vi "SN3218 Example.vi"() -> ()   [LabVIEW 2020]
uses:
  <vilib>/MakerHub/LINX/Public/Utilities/Open Local.vi
  LINX I2C/LINX I2C.lvclass
  LINX-SN3218/LINX-SN3218.lvclass
  <vilib>/MakerHub/LINX/LMH-LINX.lvlib
panel:
  in  "Channel Output":u8(slide) scale=0.0..255.0
  in  "LED Channel (0-18, 0=all)":u8
  in  "Enabled?":bool[](array[boolean])=[FALSE, FALSE, FALSE, FALSE, FALSE, FALSE, FALSE, FALSE, FALSE, FALSE, FALSE, FALSE, FALSE, FALSE, FALSE, FALSE, FALSE, FALSE]
  in  "stop":bool
  out "Error Out":errorcluster
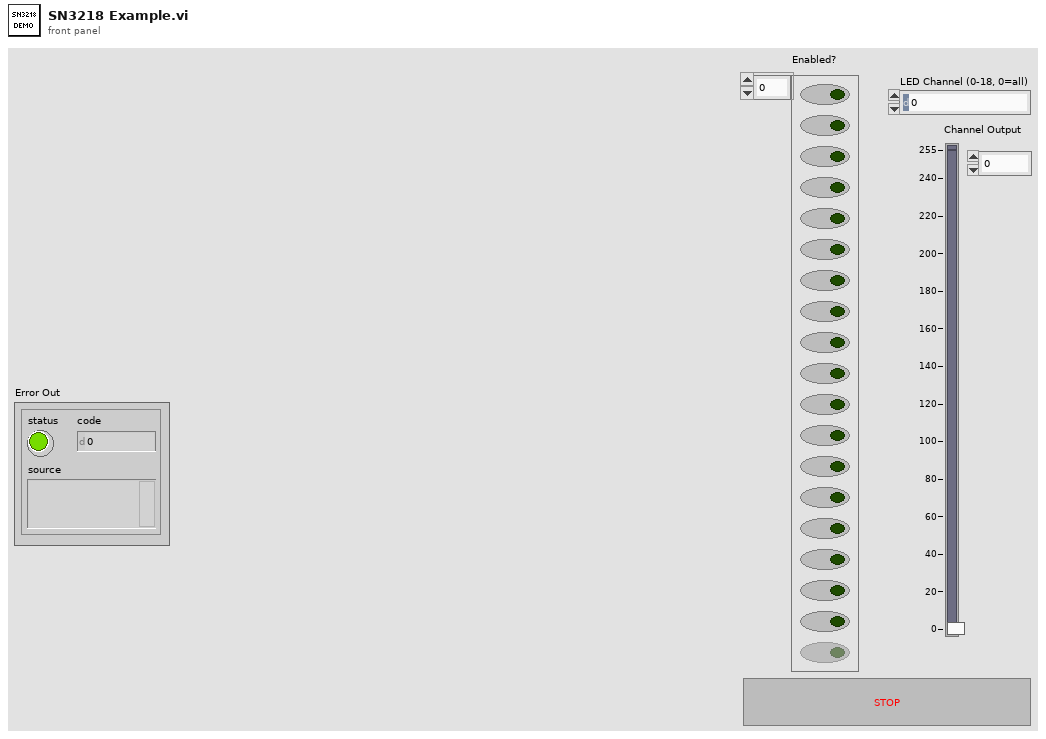
[diagram p1: front panel]
types:
  T1 = typedef "LMH-LINX.lvlib/LINX Ref.ctl" = cluster{"IO":T2, "Interface":T3, "LINX Device Config":T4}
  T2 = typedef "LMH-LINX.lvlib/Platform.ctl" = enum16{"Remote", "Local"}
  T3 = typedef "LMH-LINX.lvlib/Interface.ctl" = enum16{"Serial", "TCP"}
  T4 = typedef "LMH-LINX.lvlib/Device.lvlib/LINX Device Config.ctl" = cluster{"Interface":T3, "COM Port":refnum<visa-resource-name>, "TCP Configuration":T5, "Device Family":u8, "Device ID":u8, "Device Name":string, "TCP Ref":refnum<k5>, "Channels":T6}
  T5 = typedef "LMH-LINX.lvlib/Device.lvlib/TCP Config.ctl" = cluster{"IP Address":string, "Port":u16}
  T6 = typedef "LMH-LINX.lvlib/Channels.ctl" = cluster{"DI":u8[], "DO":u8[], "AI":u8[], "AO":u8[], "PWM":u8[], "QE":u8[], "UART":u8[], "I2C 2":u8[], "SPI":u8[], "CAN":u8[], "Servo":u8[], "AI Ref (V)":dbl, "AI Resolution (Bits)":u8, "AO Ref (V)":dbl, "AO Resolution (Bits)":u8}
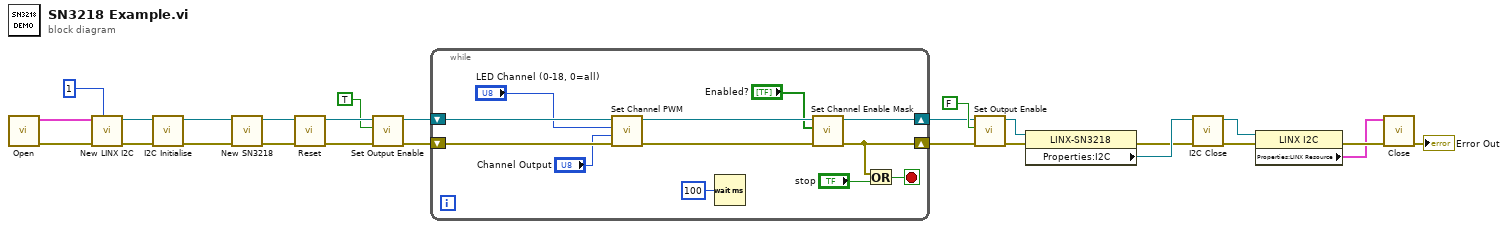
[diagram p0: block diagram]
diagram:
  n1 = call-poly <vilib>:"Open.vi"() -> ("Error Out"=w24:errorcluster, "LINX Resource"=w25:T1)  [unwired: 9 in, 1 out]
  n2 = call "New LINX I2C.vi"("LINX I2C Channel"=u8 1 ("I2C Channel"), "error in (no error)"=w24, "LINX Resource"=w25) -> ("error out"=w22:errorcluster, "LINX I2C out"=w21:refnum<class "LINX I2C.lvclass">)  [unwired: 7 in]
  n3 = call-dynamic "I2C Initialise.vi"("error in (no error)"=w22, "LINX I2C in"=w21) -> ("error out"=w14:errorcluster, "LINX I2C out"=w13:refnum<class "LINX I2C.lvclass">)  [unwired: 8 in]
  n4 = call "New SN3218.vi"("error in (no error)"=w14, "I2C"=w13) -> ("error out"=w12:errorcluster, "LINX-SN3218 out"=w11:refnum<class "LINX-SN3218.lvclass">)  [unwired: 8 in]
  n5 = call "Reset.vi"("error in (no error)"=w12, "LINX-SN3218 in"=w11) -> ("error out"=w10:errorcluster, "LINX-SN3218 out"=w9:refnum<class "LINX-SN3218.lvclass">)  [unwired: 8 in]
  n6 = call "Set Output Enable.vi"("error in (no error)"=w10, "Enabled?"=TRUE, "LINX-SN3218 in"=w9) -> ("error out"=w4:errorcluster, "LINX-SN3218 out"=w3:refnum<class "LINX-SN3218.lvclass">)  [unwired: 7 in]
  n7 = while {
    shift-right: [w35] -> w1
    shift-left: w3 -> [w33]
    shift-right: [w34] -> w2
    shift-left: w4 -> [w30]
    stop <- w38 stop-if-true
    n8 = call "Set Channel PWM.vi"("error in (no error)"=w30, "PWM (0-255)"="Channel Output", "LED Channel (0-18, 0=all)"="LED Channel (0-18, 0=all)", "LINX-SN3218 in"=w33) -> ("error out"=w31:errorcluster, "LINX-SN3218 out"=w32:refnum<class "LINX-SN3218.lvclass">)  [unwired: 6 in]
    n9 = Wait (ms)(milliseconds to wait=u32 100) -> ()  [unwired: 1 out]
    n10 = call "Set Channel Enable Mask.vi"("error in (no error)"=w31, "Channel Enable"="Enabled?", "LINX-SN3218 in"=w32) -> ("error out"=w34:errorcluster, "LINX-SN3218 out"=w35:refnum<class "LINX-SN3218.lvclass">)  [unwired: 7 in]
    n11 = Or(x=w34, y="stop") -> (x .or. y?=w38:bool)
  }
  n12 = call "Set Output Enable.vi"("error in (no error)"=w2, "Enabled?"=FALSE, "LINX-SN3218 in"=w1) -> ("error out"=w7:errorcluster, "LINX-SN3218 out"=w6:refnum<class "LINX-SN3218.lvclass">)  [unwired: 7 in]
  n13 = property class="LINX-SN3218"(reference=w6, error in=w7) -> (error out=w19:errorcluster, "Properties:I2C"=w20:refnum<class "LINX I2C.lvclass">)  [unwired: 1 out]
  n14 = call-dynamic "I2C Close.vi"("error in (no error)"=w19, "LINX I2C in"=w20) -> ("error out"=w18:errorcluster, "LINX I2C out"=w16:refnum<class "LINX I2C.lvclass">)  [unwired: 8 in]
  n15 = property class="LINX I2C"(reference=w16, error in=w18) -> (error out=w17:errorcluster, "Properties:LINX Resource"=w15:T1)  [unwired: 1 out]
  n16 = call <vilib>:"Close.vi"("Error In"=w17, "LINX Resource"=w15) -> ("Error Out"=→"Error Out":errorcluster)  [unwired: 9 in]
